vi "circle_target.vi"(8 "y0":dbl, 9 "x0":dbl, 10 "Radius":dbl, 11 "Pixels":i32) -> (1 "Target plots":cluster{dbl[], dbl[]}[](array[cluster]))   [LabVIEW 2010]
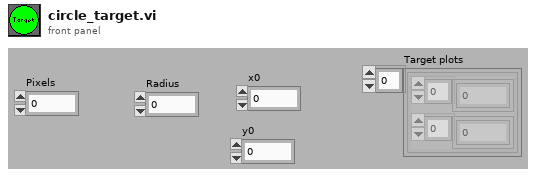
[diagram p1: front panel]
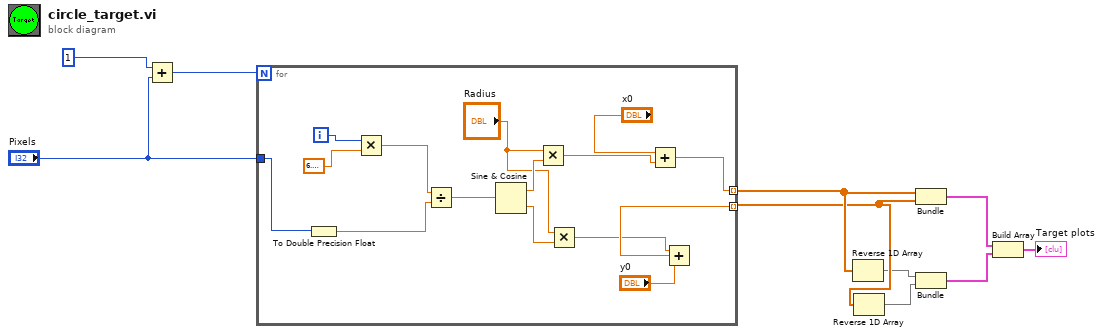
[diagram p0: block diagram]
diagram:
  n1 = Add(x=1 ("y"), y="Pixels") -> (x+y=w10:i32)
  n2 = for {
    N: w10 -> [_]
    tunnel: [w14] -> w7 mode=indexing
    tunnel: [w21] -> w6 mode=indexing
    tunnel: "Pixels" -> [w20]
    i -> [w25]
    n3 = To Double Precision Float(number=w20) -> (double precision float=w19:dbl)
    n4 = Multiply(x=w25, y=6.283185307179586) -> (x*y=w23:dbl)
    n5 = Divide(x=w23, y=w19) -> (x/y=w22:dbl)
    n6 = Sine & Cosine(0:w22) -> (1:w16:dbl, 2:w12:dbl)
    n7 = Multiply(x="Radius", y=w16) -> (x*y=w15:dbl)
    n8 = Multiply(x="Radius", y=w12) -> (x*y=w11:dbl)
    n9 = Add(x="x0", y=w15) -> (x+y=w14:dbl)
    n10 = Add(x=w11, y="y0") -> (x+y=w21:dbl)
  }
  n11 = Reverse 1D Array(array=w7) -> (reversed array=w5:dbl[])
  n12 = Reverse 1D Array(array=w6) -> (reversed array=w4:dbl[])
  n13 = Bundle(w7, w6) -> (w1:cluster{dbl[], dbl[]})  [unwired: 1 in]
  n14 = Bundle(w5, w4) -> (w3:cluster{dbl[], dbl[]})  [unwired: 1 in]
  n15 = Build Array(w1, w3) -> (→"Target plots":cluster{dbl[], dbl[]}[])
